vi "zadanie_1.vi"() -> ()   [LabVIEW 2020]
uses:
  <vilib>/express/express arith-compare/Formula/XNode/ExpressFormulaBlockNode.xnode
panel:
  in  "stop":bool
  out "Result":dbl
  out "Numeric 4":dbl caption="Xmax"
  out "Numeric 3":dbl caption="Xmin"
  out "XY Graph":cluster{"Y":dbl[], "Y":dbl[]}[](graph)
  in  "Boolean":bool caption="Wartosc bezwzgledna"
  in  "Numeric 2":dbl caption="Xmax"
  in  "Numeric":dbl caption="Xmin"
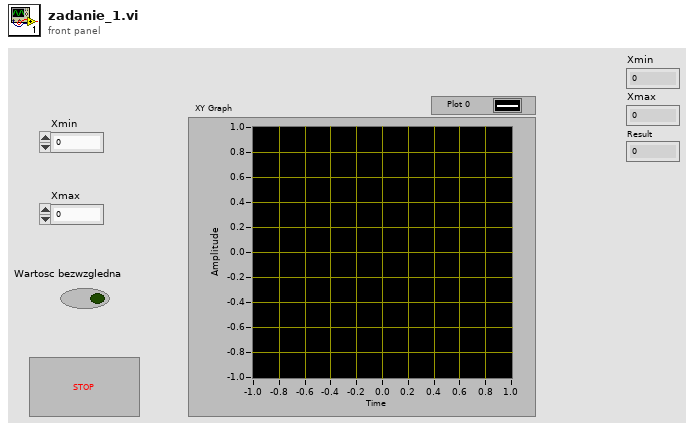
[diagram p1: front panel]
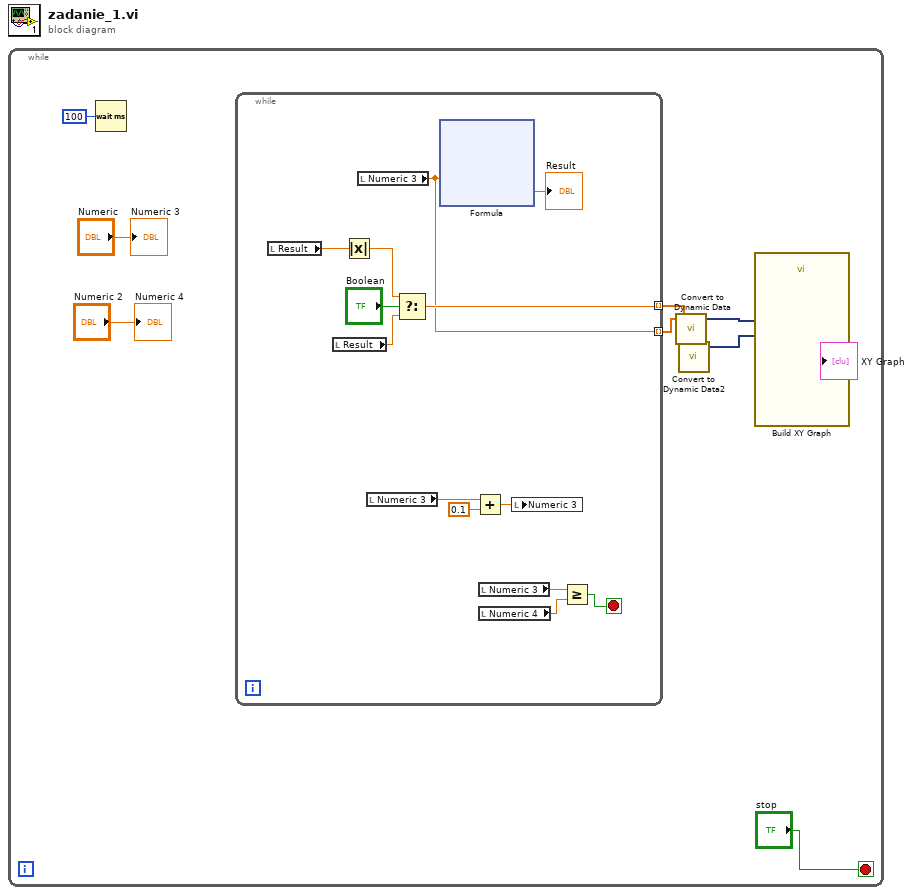
[diagram p0: block diagram]
diagram:
  n1 = while {
    stop <- "stop" stop-if-true
    n2 = Wait (ms)(milliseconds to wait=u32 100) -> ()  [unwired: 1 out]
    n3 = while {
      tunnel: [w11] -> w5 mode=indexing
      tunnel: [w10] -> w4 mode=indexing
      stop <- w12 stop-if-true
      n4 = local read "Result"() -> (w13:dbl)
      n5 = local read "Result"() -> (w15:dbl)
      n6 = Absolute Value(x=w13) -> (abs(x)=w14:dbl)
      n7 = local read "Numeric 3"() -> (w10:dbl)
      n8 = local read "Numeric 3"() -> (w22:dbl)
      n9 = Select(t=w14, s="Boolean", f=w15) -> (s? t:f=w11:dbl)
      n10 = xnode "Formula"("X1"=w10) -> ("Result"=→"Result":dbl)  [unwired: 1 in, 1 out]
      n11 = Add(x=w22, y=0.1) -> (x+y=w20:dbl)
      n12 = local read "Numeric 3"() -> (w19:dbl)
      n13 = local read "Numeric 4"() -> (w18:dbl)
      n14 = local write "Numeric 3"(w20) -> ()
      n15 = Greater Or Equal?(x=w19, y=w18) -> (x >= y?=w12:bool)
    }
    n16 = call "Convert to Dynamic Data"("Array"=w4) -> ("Dynamic Data Type"=w3:dynamicdata)  [unwired: 3 in]
    n17 = call "Convert to Dynamic Data2"("Array"=w5) -> ("Dynamic Data Type"=w2:dynamicdata)  [unwired: 3 in]
    n18 = call "Build XY Graph"("Y Input"=w2, "X Input"=w3) -> ("XY Graph"=→"XY Graph":cluster{"X":dbl[], "Y":dbl[]}[])  [unwired: 8 in, 1 out]
    "Numeric 3" <- "Numeric"
    "Numeric 4" <- "Numeric 2"
  }
